vi "PWM Output Post Step Type.vi"(8 "error in (no error)":errorcluster, 9 "PWM Output In":T1, 10 "Socket No":u16=1, 11 "PWM Output in":refnum<class "PWM Output.lvclass">) -> (0 "error out":errorcluster, 3 "PWM Output out":refnum<class "PWM Output.lvclass">)   [LabVIEW 2023, in "HardwareAbstractionLayer_LVOOP.lvlib" / "PWM Output.lvclass"]
uses:
  PWM Output.lvclass
  NI PWM Output_class/NI PWM DAQ/Control/PWM Output Edit.ctl
  NI PWM Output_class/NI PWM Output.lvclass
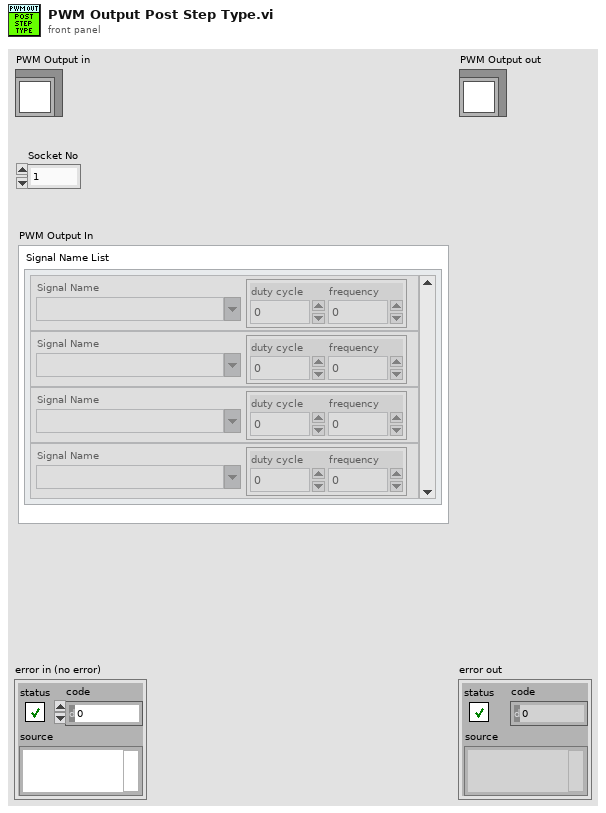
[diagram p1: front panel]
types:
  T1 = typedef "HardwareAbstractionLayer_LVOOP.lvlib/NI PWM Output.lvclass/PWM Output Edit.ctl" = cluster{"Signal Name List":cluster{"Signal Name":string, "values":cluster{"duty cycle":dbl, "frequency":dbl}}[]}
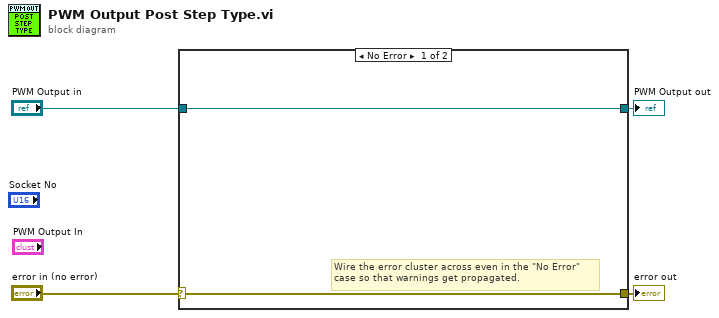
[diagram p0: block diagram]
diagram:
  n1 = case shown="No Error" "error in (no error)" {
    selector: "error in (no error)" -> [w6 w8]
    tunnel: [w6 w8] -> w3
    tunnel: [w5 w7] -> w1
    tunnel: "PWM Output in" -> [w5 w7]
    frame No Error {
      # "Wire the error cluster across even in the \"No Error\"\ncase so that warnings get propagated."
    }
    frame Error {
    }
  }
  "error out" <- w3
  "PWM Output out" <- w1
